vi "CRC4.vi"(4 "Correction Values":u16[](array[numeric])=[12594, 13108, 13622, 14136, 14656, 16706, 17220, 17664] format="%x") -> (1 "Pass CRC?":bool)   [LabVIEW 2014]
doc: "This VI computes a CRC16 checksum from <B>message</B>.\nFor compatibility with the MODbus protocol the hi and low bytes of the CRC are swapped."
panel:
  out "appended array":u16[](array[numeric]) format="%x"
  out "CRC4":u16 format="%x"
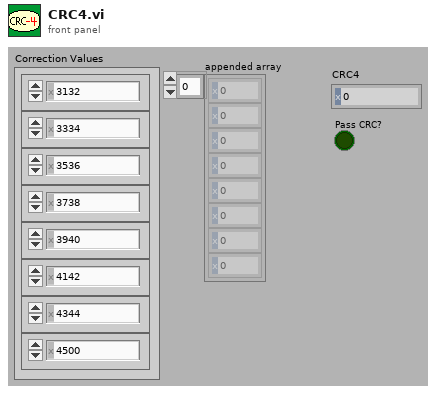
[diagram p1: front panel]
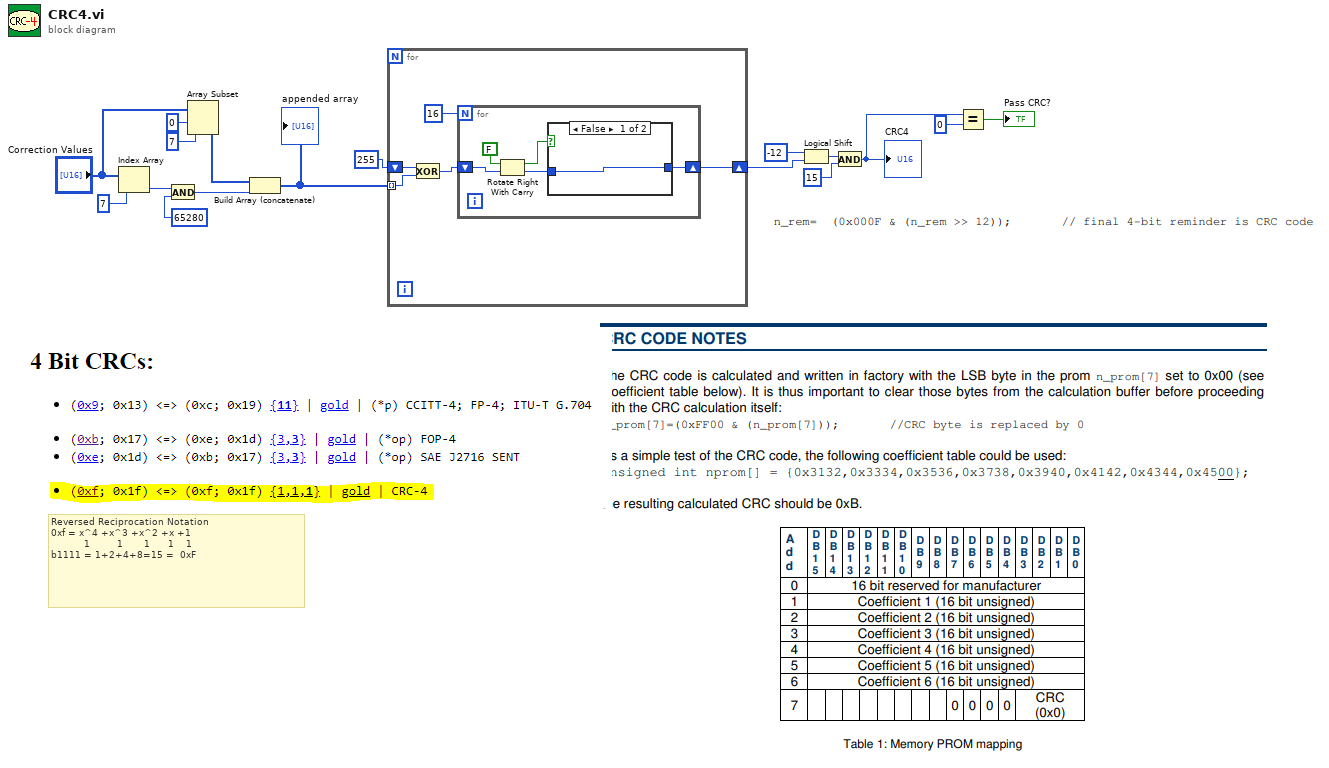
[diagram p0: block diagram]
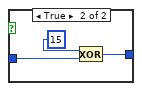
[diagram p2: hidden frame]
diagram:
  # "Reversed Reciprocation Notation\n0xf = x^4 +x^3 +x^2 +x +1\n           1         1       1      1    1\nb1111 = 1+2+4+8=15 =  0xF"
  n1 = Index Array(array="Correction Values", index=7) -> (element=w8:u16)
  n2 = And(x=w8, y=u16 65280) -> (x .and. y?=w9:u16)
  n3 = Array Subset(array="Correction Values", index=0, length=7) -> (w10:u16[])
  n4 = Build Array (concatenate)(w10, w9) -> (w12:u16[])
  "appended array" <- w12
  n5 = for {
    shift-right: [w21] -> w7
    shift-left: u16 255 -> [w20]
    tunnel: w12 -> [w19] mode=indexing
    n6 = Exclusive Or(1:w19, 2:w20) -> (0:w18:u16)
    n7 = for {
      N: 16 -> [_]
      shift-right: [w26] -> w21
      shift-left: w18 -> [w25]
      n8 = Rotate Right With Carry(2:w25, 3:FALSE ("Übertrag")) -> (0:w27:u16, 1:w24:bool)
      n9 = case shown="False" w24 {
        tunnel: w27 -> [w28 w31]
        tunnel: [w28 w30] -> w26
        frame False {
        }
        frame True {
          n10 = Exclusive Or(1:w31, 2:u8 15 ("x")) -> (0:w30:u16)
        }
      }
    }
  }
  n11 = Logical Shift(y=i16 -12, x=w7) -> (x << y=w5:u16)
  n12 = And(x=w5, y=u16 15) -> (x .and. y?=w2:u16)
  "CRC4" <- w2
  n13 = Equal?(x=w2, y=u16 0) -> (x = y?=→"Pass CRC?":bool)
